vi "Surface_modularity_Sub.vi"(5 "Y Position":string, 6 "X Position":string, 7 "Roughness Density":string="6.25", 8 "Roughness Pattern":string="Staggered") -> (3 "Output values":string[][](array[string]))   [LabVIEW 2010]
panel:
  # "Modular X Position"
  # "Modular Y Position"
  # "Module Element"
  # "Module Centre"
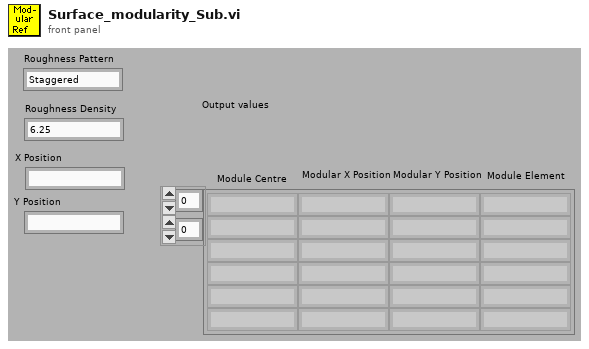
[diagram p1: front panel]
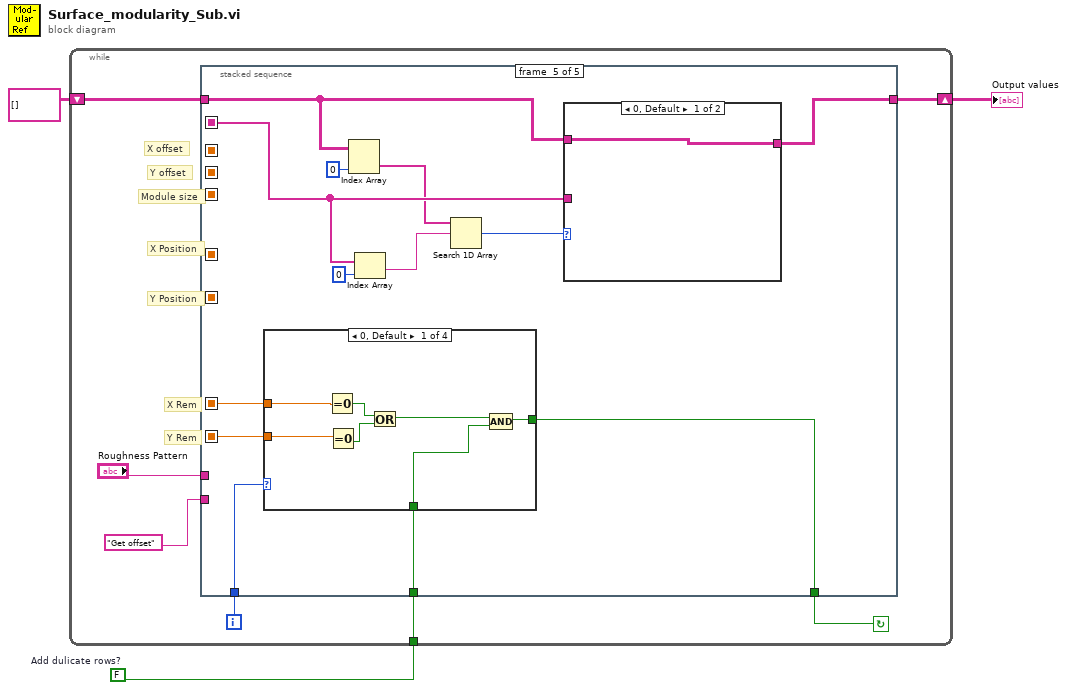
[diagram p0: block diagram]
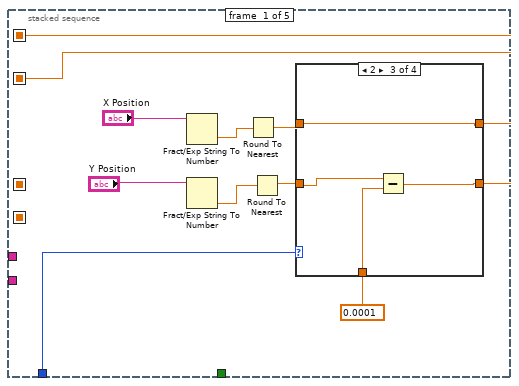
[diagram p2: hidden frame]
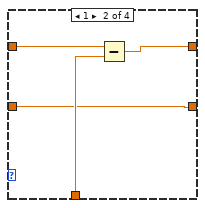
[diagram p4: hidden frame]
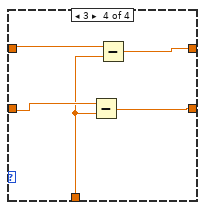
[diagram p5: hidden frame]
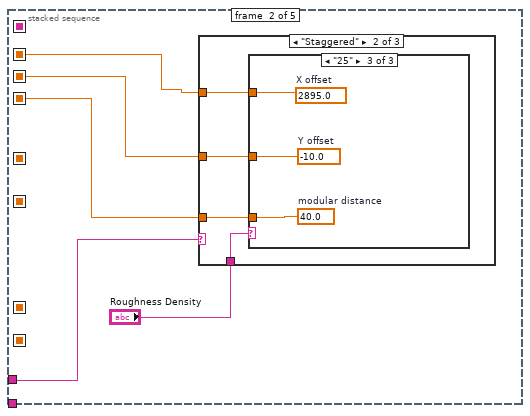
[diagram p6: hidden frame]
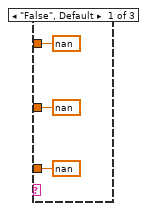
[diagram p7: hidden frame]
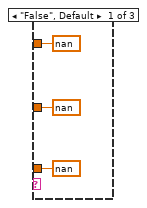
[diagram p8: hidden frame]
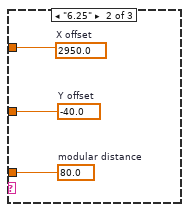
[diagram p9: hidden frame]
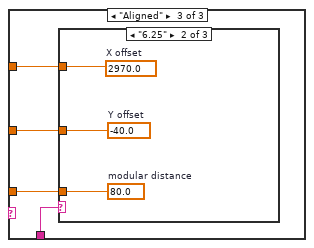
[diagram p10: hidden frame]
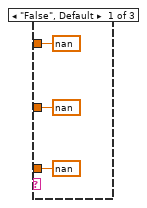
[diagram p11: hidden frame]
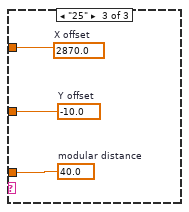
[diagram p12: hidden frame]
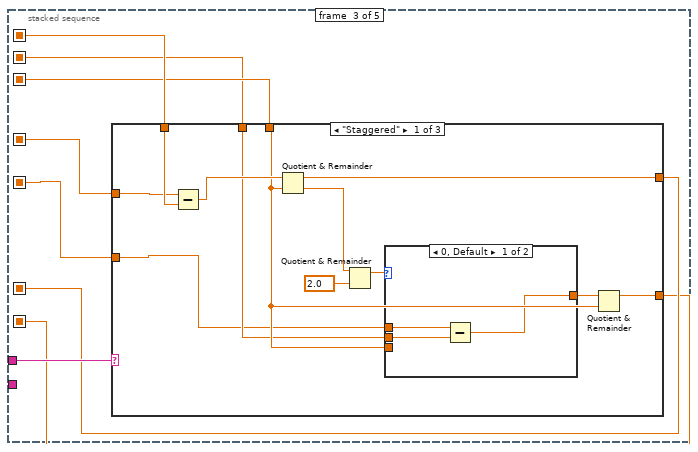
[diagram p13: hidden frame]
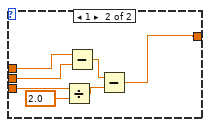
[diagram p14: hidden frame]
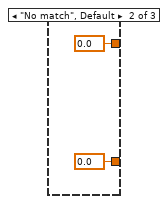
[diagram p15: hidden frame]
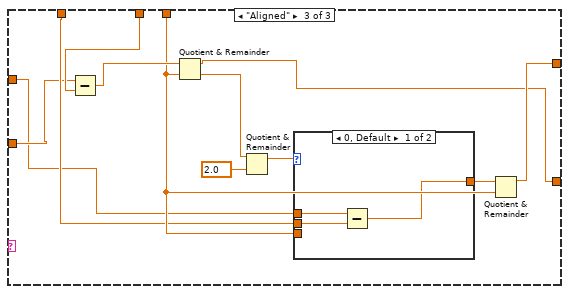
[diagram p16: hidden frame]
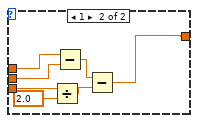
[diagram p17: hidden frame]
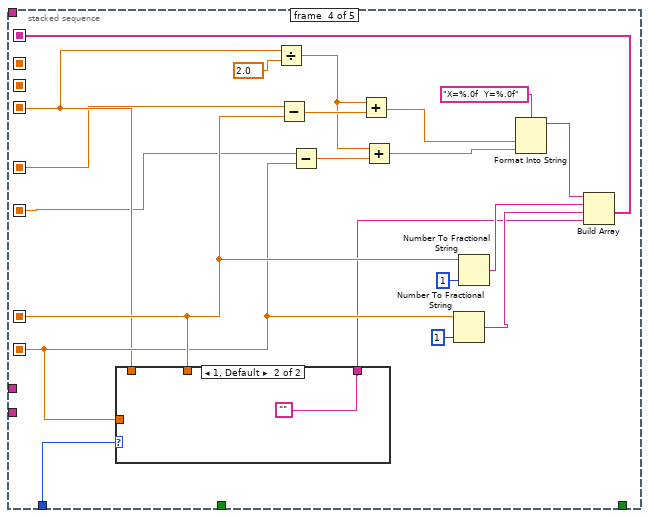
[diagram p18: hidden frame]
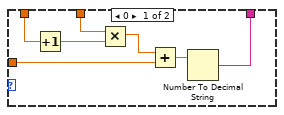
[diagram p19: hidden frame]
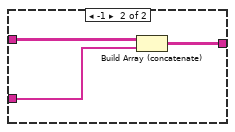
[diagram p20: hidden frame]
diagram:
  w1 = FALSE  # Add dulicate rows?
  n1 = while {
    shift-right: [w5] -> w3
    shift-left: string[][] [] -> [w6]
    tunnel: w1 -> [w4]
    i -> [w8]
    stop <- w7 continue-if-true
    # "Y Position"
    # "X Position"
    # "Module size"
    # "Y Rem"
    # "X Rem"
    # "Y offset"
    # "X offset"
    n2 = stacked-sequence {
      seq-local: [_ w40 _ _ _] -> [_ _ w77 _ _]
      seq-local: [_ w39 _ _ _] -> [_ _ w72 _ _]
      seq-local: [_ w38 _ _ _] -> [_ _ w73 w134 _]
      seq-local: [_ _ w75 _ _] -> [_ _ _ w140 w163]
      seq-local: [_ _ w74 _ _] -> [_ _ _ w139 w164]
      seq-local: [_ _ _ w127 _] -> [_ _ _ _ w157]
      seq-local: [w19 _ _ _ _] -> [_ _ w71 w126 _]
      seq-local: [w18 _ _ _ _] -> [_ _ w70 w125 _]
      tunnel: "Get offset" -> [_ _ _ _ _]
      tunnel: "Roughness Pattern" -> [_ w37 w76 _ _]
      tunnel: w8 -> [w20 _ _ w124 w162]
      tunnel: [_ _ _ _ w161] -> w7
      tunnel: w6 -> [_ _ _ _ w160]
      tunnel: [_ _ _ _ w159] -> w5
      tunnel: w4 -> [_ _ _ _ w152]
      frame #0 {
        n3 = Fract/Exp String To Number(string="X Position") -> (number=w14:dbl)  [unwired: 4 out]
        n4 = Fract/Exp String To Number(string="Y Position") -> (number=w13:dbl)  [unwired: 4 out]
        n5 = Round To Nearest(number=w14) -> (nearest integer value=w16:dbl)
        n6 = Round To Nearest(number=w13) -> (nearest integer value=w11:dbl)
        n7 = case shown="2" w20 {
          tunnel: [w22 w24 w27 w31] -> w19
          tunnel: w16 -> [w22 w26 w27 w33]
          tunnel: [w21 w23 w29 w35] -> w18
          tunnel: w11 -> [w21 w23 w28 w34]
          tunnel: 0.0001 ("y") -> [_ w25 w30 w32]
          frame 0, Default {
          }
          frame 1 {
            n8 = Subtract(x=w26, y=w25) -> (x-y=w24:dbl)
          }
          frame 2 {
            n9 = Subtract(x=w28, y=w30) -> (x-y=w29:dbl)
          }
          frame 3 {
            n10 = Subtract(x=w34, y=w32) -> (x-y=w35:dbl)
            n11 = Subtract(x=w33, y=w32) -> (x-y=w31:dbl)
          }
        }
      }
      frame #1 {
        n12 = case shown="\"Staggered\"" w37 {
          tunnel: [nan ("X offset") w47 w60] -> w40
          tunnel: [nan ("Y offset") w46 w59] -> w39
          tunnel: [nan ("modular distance") w45 w58] -> w38
          tunnel: "Roughness Density" -> [_ w44 w57]
          frame "False", Default {
          }
          frame "Staggered" {
            n13 = case shown="\"25\"" w44 {
              tunnel: [nan ("X offset") w53 w56] -> w47
              tunnel: [nan ("Y offset") w52 w55] -> w46
              tunnel: [nan ("modular distance") w51 w54] -> w45
              frame "False", Default {
              }
              frame "6.25" {
                w51 = 80.0  # modular distance
                w52 = -40.0  # Y offset
                w53 = 2950.0  # X offset
              }
              frame "25" {
                w54 = 40.0  # modular distance
                w55 = -10.0  # Y offset
                w56 = 2895.0  # X offset
              }
            }
          }
          frame "Aligned" {
            n14 = case shown="\"6.25\"" w57 {
              tunnel: [nan ("X offset") w66 w69] -> w60
              tunnel: [nan ("Y offset") w65 w68] -> w59
              tunnel: [nan ("modular distance") w64 w67] -> w58
              frame "False", Default {
              }
              frame "6.25" {
                w64 = 80.0  # modular distance
                w65 = -40.0  # Y offset
                w66 = 2970.0  # X offset
              }
              frame "25" {
                w67 = 40.0  # modular distance
                w68 = -10.0  # Y offset
                w69 = 2870.0  # X offset
              }
            }
          }
        }
      }
      frame #2 {
        n15 = case shown="\"Staggered\"" w76 {
          tunnel: w73 -> [w84 _ w108]
          tunnel: w77 -> [w83 _ w106]
          tunnel: w72 -> [w82 _ w107]
          tunnel: w71 -> [w81 _ w104]
          tunnel: w70 -> [w80 _ w105]
          tunnel: [w79 0.0 w103] -> w75
          tunnel: [w78 0.0 w102] -> w74
          frame "Staggered" {
            n16 = Subtract(x=w81, y=w83) -> (x-y=w89:dbl)
            n17 = Quotient & Remainder(x=w89, y=w84) -> (x-y*floor(x/y)=w79:dbl, floor(x/y)=w88:dbl)
            n18 = Quotient & Remainder(x=w88, y=2.0) -> (x-y*floor(x/y)=w86:dbl)  [unwired: 1 out]
            n19 = case shown="0, Default" w86 {
              tunnel: w80 -> [w92 w99]
              tunnel: w82 -> [w91 w98]
              tunnel: [w90 w93] -> w85
              tunnel: w84 -> [_ w95]
              frame 0, Default {
                n20 = Subtract(x=w92, y=w91) -> (x-y=w90:dbl)
              }
              frame 1 {
                n21 = Divide(x=w95, y=2.0) -> (x/y=w94:dbl)
                n22 = Subtract(x=w99, y=w98) -> (x-y=w97:dbl)
                n23 = Subtract(x=w97, y=w94) -> (x-y=w93:dbl)
              }
            }
            n24 = Quotient & Remainder(x=w85, y=w84) -> (x-y*floor(x/y)=w78:dbl)  [unwired: 1 out]
          }
          frame "No match", Default {
          }
          frame "Aligned" {
            n25 = Subtract(x=w105, y=w107) -> (x-y=w113:dbl)
            n26 = Quotient & Remainder(x=w113, y=w108) -> (x-y*floor(x/y)=w102:dbl, floor(x/y)=w112:dbl)
            n27 = Quotient & Remainder(x=w112, y=2.0) -> (x-y*floor(x/y)=w110:dbl)  [unwired: 1 out]
            n28 = case shown="0, Default" w110 {
              tunnel: w104 -> [w116 w123]
              tunnel: w106 -> [w115 w122]
              tunnel: [w114 w117] -> w109
              tunnel: w108 -> [_ w119]
              frame 0, Default {
                n29 = Subtract(x=w116, y=w115) -> (x-y=w114:dbl)
              }
              frame 1 {
                n30 = Divide(x=w119, y=2.0) -> (x/y=w118:dbl)
                n31 = Subtract(x=w123, y=w122) -> (x-y=w121:dbl)
                n32 = Subtract(x=w121, y=w118) -> (x-y=w117:dbl)
              }
            }
            n33 = Quotient & Remainder(x=w109, y=w108) -> (x-y*floor(x/y)=w103:dbl)  [unwired: 1 out]
          }
        }
      }
      frame #3 {
        n34 = case shown="1, Default" w124 {
          tunnel: w140 -> [w149 _]
          tunnel: w139 -> [w148 _]
          tunnel: [w146 ""] -> w136
          tunnel: w134 -> [w145 _]
          frame 0 {
            n35 = Increment(x=w145) -> (x+1=w144:dbl)
            n36 = Multiply(x=w149, y=w144) -> (x*y=w150:dbl)
            n37 = Add(x=w150, y=w148) -> (x+y=w147:dbl)
            n38 = Number To Decimal String(number=w147) -> (decimal integer string=w146:string)  [unwired: 1 out]
          }
          frame 1, Default {
          }
        }
        n39 = Divide(x=w134, y=2.0) -> (x/y=w131:dbl)
        n40 = Subtract(x=w126, y=w140) -> (x-y=w135:dbl)
        n41 = Subtract(x=w125, y=w139) -> (x-y=w130:dbl)
        n42 = Add(x=w131, y=w135) -> (x+y=w132:dbl)
        n43 = Add(x=w131, y=w130) -> (x+y=w129:dbl)
        n44 = Number To Fractional String(number=w139, precision (6)=i16 1) -> (F-format string=w137:string)  [unwired: 2 out]
        n45 = Number To Fractional String(number=w140, precision (6)=i16 1) -> (F-format string=w138:string)  [unwired: 2 out]
        n46 = Format Into String(format string="X=%.0f  Y=%.0f", w132, w129) -> (resulting string=w128:string)  [unwired: 2 in, 1 out]
        n47 = Build Array(w128, w138, w137, w136) -> (w127:string[])
      }
      frame #4 {
        n48 = case shown="0, Default" w162 {
          tunnel: w164 -> [w175 _ _ _]
          tunnel: w163 -> [w174 _ _ _]
          tunnel: [w171 TRUE TRUE FALSE] -> w161
          tunnel: w152 -> [w169 _ _ _]
          frame 0, Default {
            n49 = Equal To 0?(x=w174) -> (x = 0?=w172:bool)
            n50 = Equal To 0?(x=w175) -> (x = 0?=w173:bool)
            n51 = Or(x=w172, y=w173) -> (x .or. y?=w170:bool)
            n52 = Compound Arithmetic op=AND(w170, w169) -> (w171:bool)
          }
          frame 1 {
          }
          frame 2 {
          }
          frame 3 {
          }
        }
        n53 = Index Array(array=w160, index (col)=0 ("disabled index (col)")) -> (element=w154:string[])  [unwired: 1 in]
        n54 = Index Array(array=w157, index=0) -> (element=w155:string)
        n55 = Search 1D Array(1D array=w154, element=w155) -> (index of element=w153:i32)  [unwired: 1 out]
        n56 = case shown="0, Default" w153 {
          tunnel: w160 -> [w165 w168]
          tunnel: [w165 w167] -> w159
          tunnel: w157 -> [_ w166]
          frame 0, Default {
          }
          frame -1 {
            n57 = Build Array (concatenate)(w168, w166) -> (w167:string[][])
          }
        }
      }
    }
  }
  "Output values" <- w3
